vi "okDeviceSensors Get Sensors Count.vi"(8 "Error In":errorcluster, 11 "okDeviceSensors Refnum":refnum<k24>) -> (0 "Error Out":errorcluster, 1 "Count":i32, 3 "okDeviceSensors Refnum":refnum<k24>)   [LabVIEW 2021, in "okFrontPanelC#Wrapper.lvlib"]
uses:
  okFrontPanelC#Wrapper.lvlib
  D:/UCLA Thinkpad Google Drive/LabVIEW 2021 SP1/builds/SwissSPAD Live Distribution/Opal Kelly/C# Wrapper/v5.0.2/libFrontPanel-csharp.dll
  v5.0.2/libFrontPanel-csharp.dll
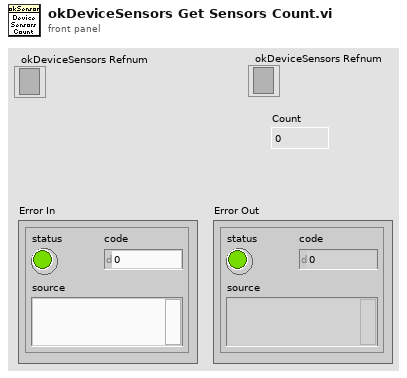
[diagram p1: front panel]
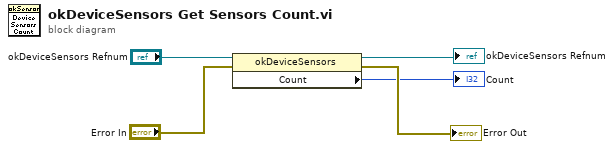
[diagram p0: block diagram]
diagram:
  n1 = property class="okDeviceSensors"(reference="okDeviceSensors Refnum", error in="Error In") -> (reference out=→"okDeviceSensors Refnum":refnum<k24>, error out=→"Error Out":errorcluster, "Count"=→"Count":i32)
